vi "整型数正则表达式（精确指定位数，单词）.vi"(8 "error in (no error)":errorcluster caption="错误输入（无错误）", 11 "位数":i32=3) -> (0 "error out":errorcluster caption="错误输出", 3 "正则表达式":string="\\d\\d\\d")   [LabVIEW 2012]
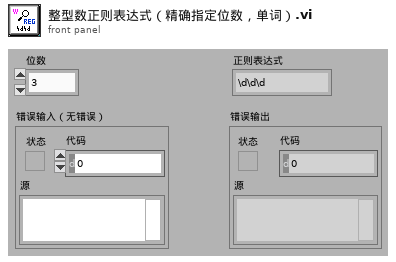
[diagram p1: front panel]
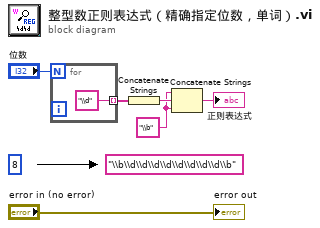
[diagram p0: block diagram]
diagram:
  (unwired) "\\b\\d\\d\\d\\d\\d\\d\\d\\d\\b" ("正则表达式")
  (unwired) 8 ("位数")
  w2 = "\\b"
  n1 = for {
    N: "位数" -> [_]
    tunnel: ["\\d"] -> w4 mode=indexing
  }
  n2 = Concatenate Strings(w4) -> (w3:string)
  n3 = Concatenate Strings(w2, w3, w2) -> (→"正则表达式":string)
  "error out" <- "error in (no error)"
